vi "TerminarPrueba.vi"(8 "error in (no error)":errorcluster, 9 "String":string, 11 "Prueba33 in":refnum<class "Prueba33.lvclass">) -> (0 "error out":errorcluster, 3 "Prueba33 out":refnum<class "Prueba33.lvclass">)   [LabVIEW 2019, in "Prueba33.lvclass"]
uses:
  Prueba33.lvclass
  Controles/Tab.ctl
  Prueba33.lvclass/Prueba33.ctl
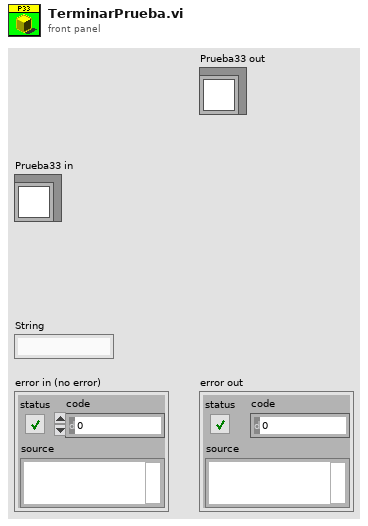
[diagram p1: front panel]
types:
  T1 = typedef "Prueba33.lvclass/Tab.ctl" = enum32{"Main", "D1_A", "D1_B", "D2_A", "D2_B", "D3_A", "D3_B", "D4_A", "D4_B"}
  T2 = cluster{"ControlName":string, "ControlReference":refnum<vi>}[]
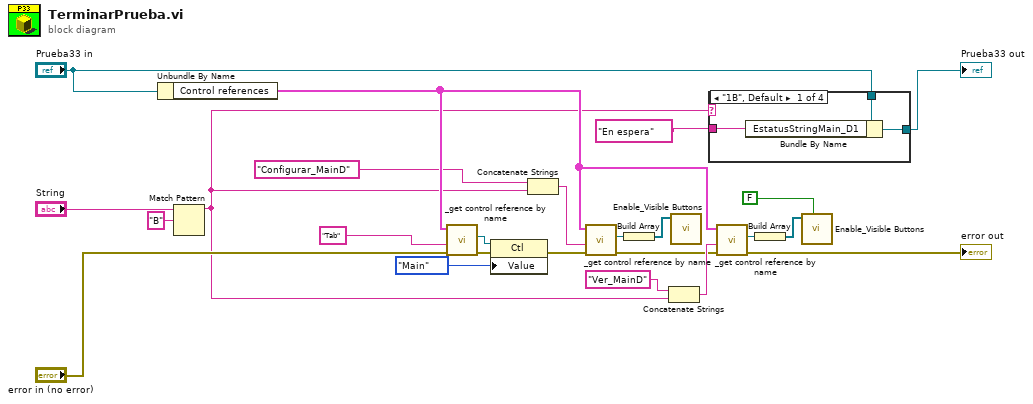
[diagram p0: block diagram]
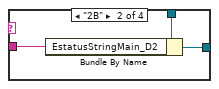
[diagram p2: hidden frame]
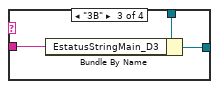
[diagram p3: hidden frame]
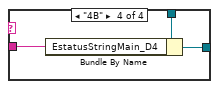
[diagram p4: hidden frame]
diagram:
  n1 = Unbundle By Name("Prueba33 in") -> ("Control references"=w24:T2)
  n2 = Match Pattern(string="String", regular expression="B") -> (before substring=w3:string)  [unwired: 1 in, 3 out]
  n3 = call "_get control reference by name.vi"("error in (no error)"="error in (no error)", "Control name"="Tab" ("Message"), "Control references"=w24) -> ("error out"=w9:errorcluster, "Ctl Refnum"=w8:refnum<vi>)  [unwired: 3 in]
  n4 = property class="Ctl"(reference=w8, error in=w9, "Value"=Tab."Main" ("Tab")) -> (error out=w22:errorcluster)  [unwired: 1 out]
  n5 = Concatenate Strings("Configurar_MainD" ("Message"), w3) -> (w2:string)
  n6 = call "_get control reference by name.vi"("error in (no error)"=w22, "Control name"=w2, "Control references"=w24) -> ("error out"=w19:errorcluster, "Ctl Refnum"=w15:refnum<vi>)  [unwired: 3 in]
  n7 = Build Array(w15) -> (w16:refnum<vi>[])
  n8 = Concatenate Strings("Ver_MainD" ("Message"), w3) -> (w20:string)
  n9 = call "Enable_Visible Buttons.vi"("Controls Ref Array"=w16) -> ()  [unwired: 11 in]
  n10 = case shown="\"1B\", Default" w3 {
    tunnel: [w27 w30 w33 w36] -> w11
    tunnel: "Prueba33 in" -> [w26 w29 w32 w35]
    tunnel: "En espera" ("Message") -> [w25 w28 w31 w34]
    frame "1B", Default {
      n11 = Bundle By Name(cluster=w26, "EstatusStringMain_D1"=w25) -> (w27:refnum<class "Prueba33.lvclass">)
    }
    frame "2B" {
      n12 = Bundle By Name(cluster=w29, "EstatusStringMain_D2"=w28) -> (w30:refnum<class "Prueba33.lvclass">)
    }
    frame "3B" {
      n13 = Bundle By Name(cluster=w32, "EstatusStringMain_D3"=w31) -> (w33:refnum<class "Prueba33.lvclass">)
    }
    frame "4B" {
      n14 = Bundle By Name(cluster=w35, "EstatusStringMain_D4"=w34) -> (w36:refnum<class "Prueba33.lvclass">)
    }
  }
  "Prueba33 out" <- w11
  n15 = call "_get control reference by name.vi"("error in (no error)"=w19, "Control name"=w20, "Control references"=w24) -> ("error out"=→"error out":errorcluster, "Ctl Refnum"=w18:refnum<vi>)  [unwired: 3 in]
  n16 = Build Array(w18) -> (w17:refnum<vi>[])
  n17 = call "Enable_Visible Buttons.vi"("Enable? (T)"=FALSE, "Controls Ref Array"=w17) -> ()  [unwired: 10 in]
